vi "ReversedEngineering ConvertTypeDefsAttributesToString.vi"(1 "TypeDef":T1, 5 "error in (no error)":errorcluster) -> (15 "className":string, 16 "attributes":string, 18 "ClassPath":path, 19 "error out":errorcluster)   [LabVIEW 2014]
uses:
  <resource>/Framework/Providers/Open_GDS/UML/ReversedEngineering/ReversedEngineering TypeDefType.ctl
  <resource>/Framework/Providers/Open_GDS/UML/ReversedEngineering/ReversedEngineering AttributeInfoType.ctl
  <resource>/Framework/Providers/Open_GDS/ClassProviders/Common/CommonVIs/CommonVIs_AttributeDataType.ctl
  <resource>/Framework/Providers/Open_GDS/UML/UMLEditor/UMLEditor_VisibilityType.ctl
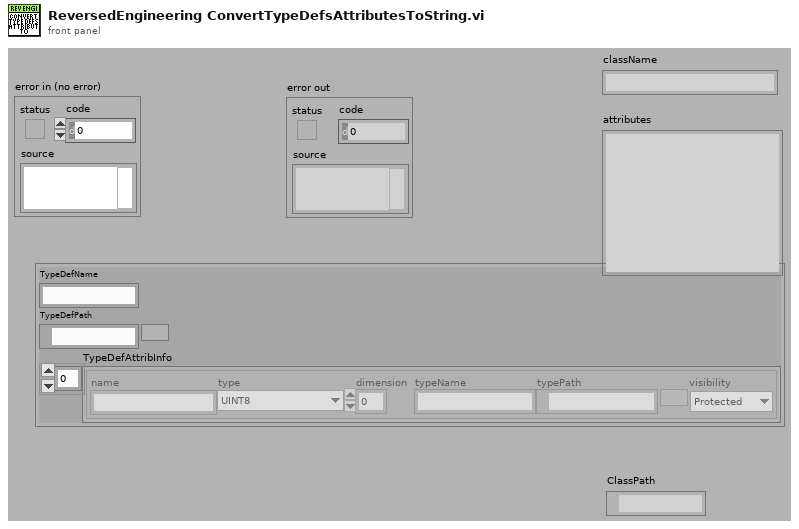
[diagram p1: front panel]
types:
  T1 = typedef "ReversedEngineering TypeDefType.ctl" = cluster{"TypeDefName":string, "TypeDefPath":path, "TypeDefAttribInfo":T2[]}
  T2 = typedef "ReversedEngineering AttributeInfoType.ctl" = cluster{"name":string, "type":T3, "dimension":i32, "typeName":string, "typePath":path, "visibility":T4}
  T3 = typedef "CommonVIs_AttributeDataType.ctl" = enum16{"UINT8", "INT8", "UINT16", "INT16", "UINT32", "INT32", "UINT64", "INT64", "SGL", "DBL", "EXT", "CSG", "CDB", "CXT", "TimeStamp", "STRING", "PATH", "BOOL", "ENUM", "RefNum", "VIRefNum", "LabVIEW Class", "Cluster", "Variant", "TypeDef", "Waveform", "LabVIEW Object", "Other", "void"}
  T4 = typedef "UMLEditor_VisibilityType.ctl" = enum16{"Public", "Private", "Protected"}
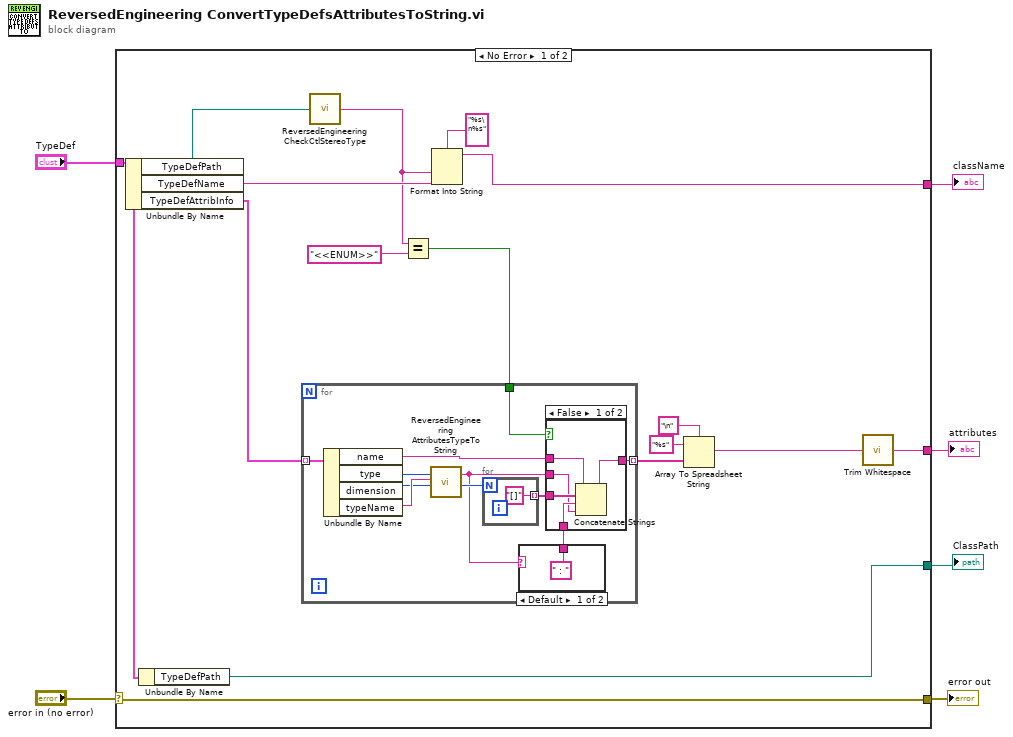
[diagram p0: block diagram]
diagram:
  n1 = case shown="No Error" "error in (no error)" {
    selector: "error in (no error)" -> [w22 w41]
    tunnel: [w22 w41] -> w6
    tunnel: "TypeDef" -> [w18 _]
    tunnel: [w8 _] -> w3
    tunnel: [w17 _] -> w2
    tunnel: [w13 _] -> w1
    frame No Error {
      n2 = Unbundle By Name(w18) -> ("TypeDefPath"=w12:path, "TypeDefName"=w14:string, "TypeDefAttribInfo"=w21:T2[])
      n3 = Unbundle By Name(w18) -> ("TypeDefPath"=w17:path)
      n4 = call <resource>:"ReversedEngineering CheckCtlStereoType.vi"("TypeDefPath"=w12) -> ("ClassDesc"=w11:string)
      n5 = Equal?(x=w11, y="<<ENUM>>" ("ClassDesc")) -> (x = y?=w9:bool)
      n6 = for {
        tunnel: w21 -> [w32] mode=indexing
        tunnel: [w25] -> w16 mode=indexing
        tunnel: w9 -> [w23]
        n7 = Unbundle By Name(w32) -> ("name"=w26:string, "type"=w31:T3, "dimension"=w29:i32, "typeName"=w30:string)
        n8 = call <resource>:"ReversedEngineering AttributesTypeToString.vi"("AttributeDataType"=w31, "name"=w30) -> ("string"=w24:string)  [unwired: 17 out]
        n9 = for {
          N: w29 -> [_]
          tunnel: ["[]"] -> w28 mode=indexing
        }
        n10 = case shown="Default" w24 {
          tunnel: [" : " _] -> w27
          frame Default {
          }
          frame "" {
          }
        }
        n11 = case shown="False" w23 {
          tunnel: w28 -> [w37 _]
          tunnel: w27 -> [w36 _]
          tunnel: w26 -> [w35 w38]
          tunnel: [w34 w38] -> w25
          tunnel: w24 -> [w33 _]
          frame False {
            n12 = Concatenate Strings(w35, w37, w36, w33) -> (w34:string)
          }
          frame True {
          }
        }
      }
      n13 = Format Into String(format string="%s\n%s", w11, w14) -> (resulting string=w13:string)  [unwired: 2 in, 1 out]
      n14 = Array To Spreadsheet String(delimiter (Tab)="\n", array=w16, 3:"%s" ("format string")) -> (spreadsheet string=w7:string)
      n15 = call <vilib>:"Trim Whitespace.vi"("string"=w7) -> ("trimmed string"=w8:string)  [unwired: 1 in]
    }
    frame Error {
    }
  }
  "error out" <- w6
  "attributes" <- w3
  "className" <- w1
  "ClassPath" <- w2
